vi "Sensor_WEB_project2.vi"() -> ()   [LabVIEW 2022 SP3]
uses:
  <vilib>/httpClient/LabVIEWHTTPClient.lvlib
panel:
  out "Control1":bool
  out "Web Address":string
  in  "Nhiet do canh bao":dbl
  out "Warning":bool
  in  "Receive Adress":string[](array[string])
  in  "API key":string
  out "Bieu do Do Am":dbl(graph)
  out "Bieu do Nhiet Do":dbl(graph)
  in  "stop":bool
  out "Do Am":dbl(slide) scale=0.0..100.0
  out "Nhiet Do":dbl(slide) scale=0.0..100.0
  in  "Port Name":refnum<visa-resource-name>
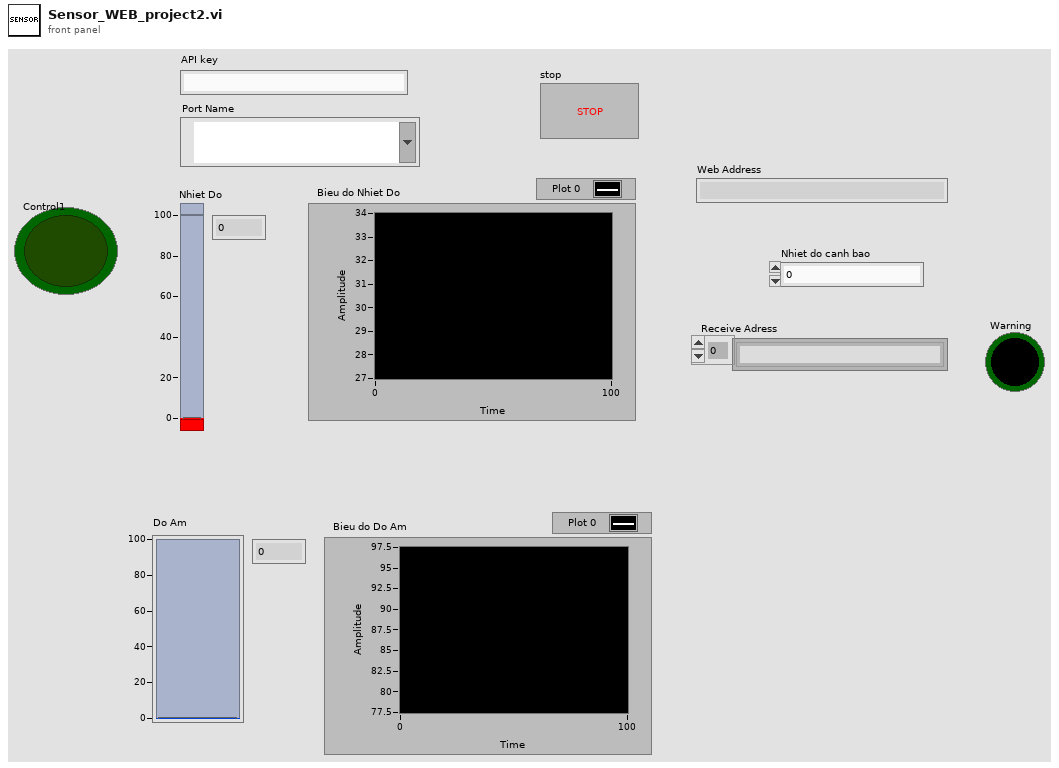
[diagram p1: front panel]
types:
  T1 = typedef "LabVIEWHTTPClient.lvlib/ClientHandle.ctl" = refnum<k1>
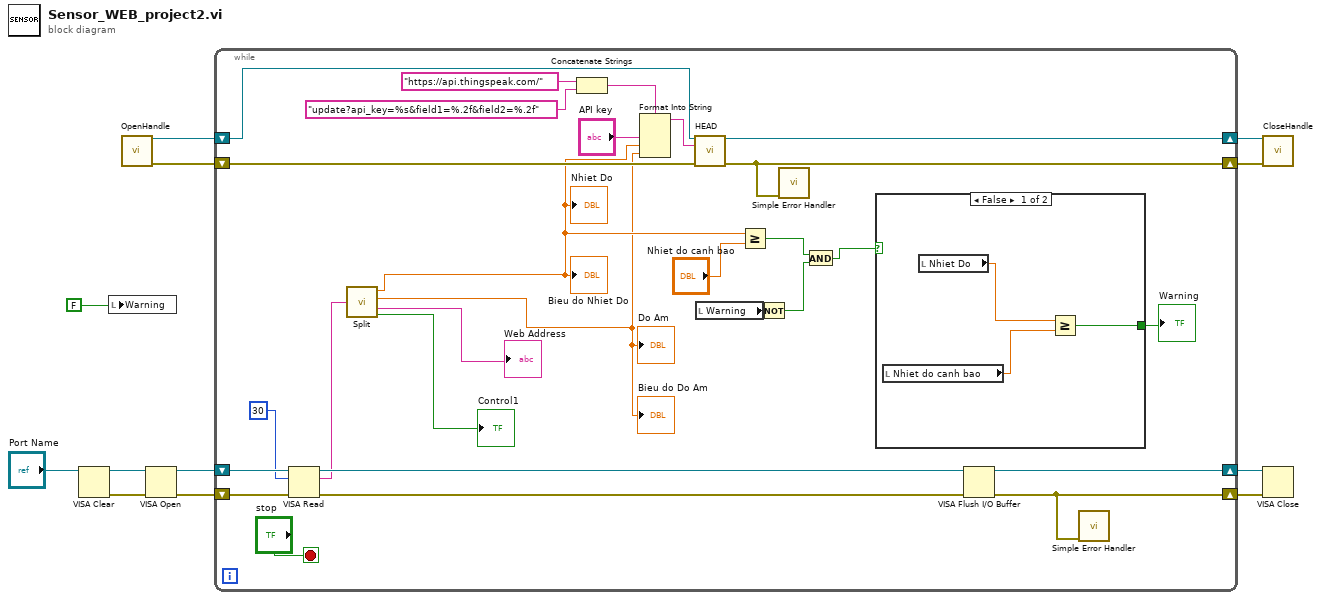
[diagram p0: block diagram]
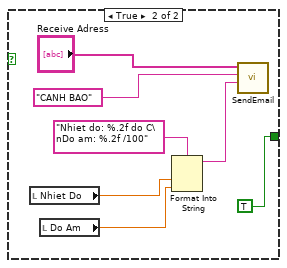
[diagram p2: hidden frame]
diagram:
  n1 = VISA Clear(VISA resource name="Port Name") -> (VISA resource name out=w12:refnum<visa-resource-name>, error out=w11:errorcluster)  [unwired: 1 in]
  n2 = local write "Warning"(FALSE) -> ()
  n3 = call <vilib>:"OpenHandle.vi"() -> ("client handle out"=w5:T1, "error out"=w4:errorcluster)  [unwired: 14 in]
  n4 = VISA Open(error in (no error)=w11, VISA resource name=w12) -> (VISA resource name=w10:refnum<visa-resource-name>, error out=w9:errorcluster)  [unwired: 3 in]
  n5 = while {
    shift-right: [w38] -> w8
    shift-left: w10 -> [w40]
    shift-right: [w18] -> w7
    shift-left: w9 -> [w39]
    shift-right: [w34] -> w3
    shift-left: w5 -> [w36]
    shift-right: [w19] -> w2
    shift-left: w4 -> [w35]
    stop <- "stop" stop-if-true
    n6 = VISA Read(VISA resource name=w40, byte count=u32 30, error in (no error)=w39) -> (VISA resource name out=w22:refnum<visa-resource-name>, read buffer=w17:string, error out=w21:errorcluster)  [unwired: 1 out]
    n7 = call "Split.vi"("INPUT STRING"=w17) -> ("temp"=w16:dbl, "humid"=w15:dbl, "Web"=→"Web Address":string, "Control1"=→"Control1":bool)
    "Nhiet Do" <- w16
    "Do Am" <- w15
    "Bieu do Nhiet Do" <- w16
    "Bieu do Do Am" <- w15
    n8 = Concatenate Strings("https://api.thingspeak.com/" ("string"), "update?api_key=%s&field1=%.2f&field2=%.2f" ("string")) -> (w31:string)
    n9 = Format Into String(format string=w31, "API key", w16, w15) -> (resulting string=w29:string)  [unwired: 2 in, 1 out]
    n10 = call <vilib>:"HEAD.vi"("client handle"=w36, "url"=w29, "error in (no error)"=w35) -> ("client handle out"=w34:T1, "error out"=w19:errorcluster)  [unwired: 10 in, 1 out]
    n11 = local read "Warning"() -> (w27:bool)
    n12 = Greater Or Equal?(x=w16, y="Nhiet do canh bao") -> (x >= y?=w26:bool)
    n13 = Not(x=w27) -> (.not. x?=w25:bool)
    n14 = call <vilib>:"Simple Error Handler.vi"("error in (no error)"=w19) -> ()  [unwired: 4 in, 5 out]
    n15 = And(x=w26, y=w25) -> (x .and. y?=w24:bool)
    n16 = case shown="False" w24 {
      tunnel: [w43 TRUE ("Boolean")] -> w28
      frame False {
        n17 = local read "Nhiet do canh bao"() -> (w41:dbl)
        n18 = local read "Nhiet Do"() -> (w42:dbl)
        n19 = Greater Or Equal?(x=w42, y=w41) -> (x >= y?=w43:bool)
      }
      frame True {
        n20 = local read "Nhiet Do"() -> (w46:dbl)
        n21 = local read "Do Am"() -> (w47:dbl)
        n22 = Format Into String(format string="Nhiet do: %.2f do C\nDo am: %.2f /100", w46, w47) -> (resulting string=w44:string)  [unwired: 2 in, 1 out]
        n23 = call "SendEmail.vi"("Body"=w44, "Subject"="CANH BAO", "Receive Adress"="Receive Adress") -> ()  [unwired: 1 in]
      }
    }
    "Warning" <- w28
    n24 = VISA Flush I/O Buffer(VISA resource name=w22, error in (no error)=w21) -> (VISA resource name out=w38:refnum<visa-resource-name>, error out=w18:errorcluster)  [unwired: 1 in]
    n25 = call <vilib>:"Simple Error Handler.vi"("error in (no error)"=w18) -> ()  [unwired: 4 in, 5 out]
  }
  n26 = call <vilib>:"CloseHandle.vi"("client handle"=w3, "error in (no error)"=w2) -> ()  [unwired: 13 in, 1 out]
  n27 = VISA Close(VISA resource name=w8, error in (no error)=w7) -> ()  [unwired: 1 out]
